vi "Connect to Slave.vi"(8 "error in (no error)":errorcluster, 11 "network master in":refnum<class "Master CR.lvclass">) -> (0 "error out":errorcluster, 3 "network master out":refnum<class "Master CR.lvclass">)   [LabVIEW 2021, in "Master CR.lvclass"]
doc: "This provides an interface for the master to open a connection to the slave."
uses:
  Master CR.lvclass
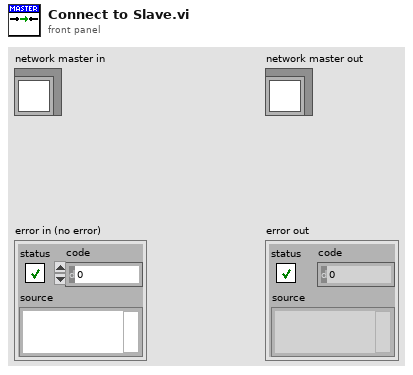
[diagram p1: front panel]
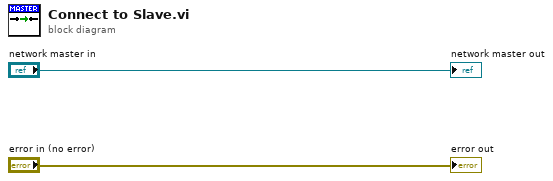
[diagram p0: block diagram]
diagram:
  "error out" <- "error in (no error)"
  "network master out" <- "network master in"
